vi "总VI.vi"() -> ()   [LabVIEW 2020]
panel:
  out "当前输入/结果":string="0"
  out "历史记录":string
  in  "=":bool
  in  ".":bool
  in  "0":bool
  in  "+/-":bool
  in  "+":bool
  in  "3":bool
  in  "2":bool
  in  "1":bool
  in  "-":bool
  in  "6":bool
  in  "5":bool
  in  "4":bool
  in  "*":bool
  in  "9":bool
  in  "8":bool
  in  "7":bool
  in  "/":bool
  in  "平方根":bool
  in  "x^2":bool
  in  "1/x":bool
  in  "回删":bool
  in  "清空全部":bool
  in  "清除输入":bool
  in  "%":bool
  # "标准"
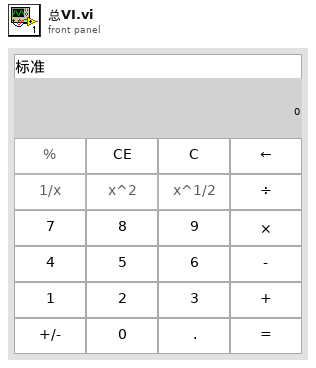
[diagram p1: front panel]
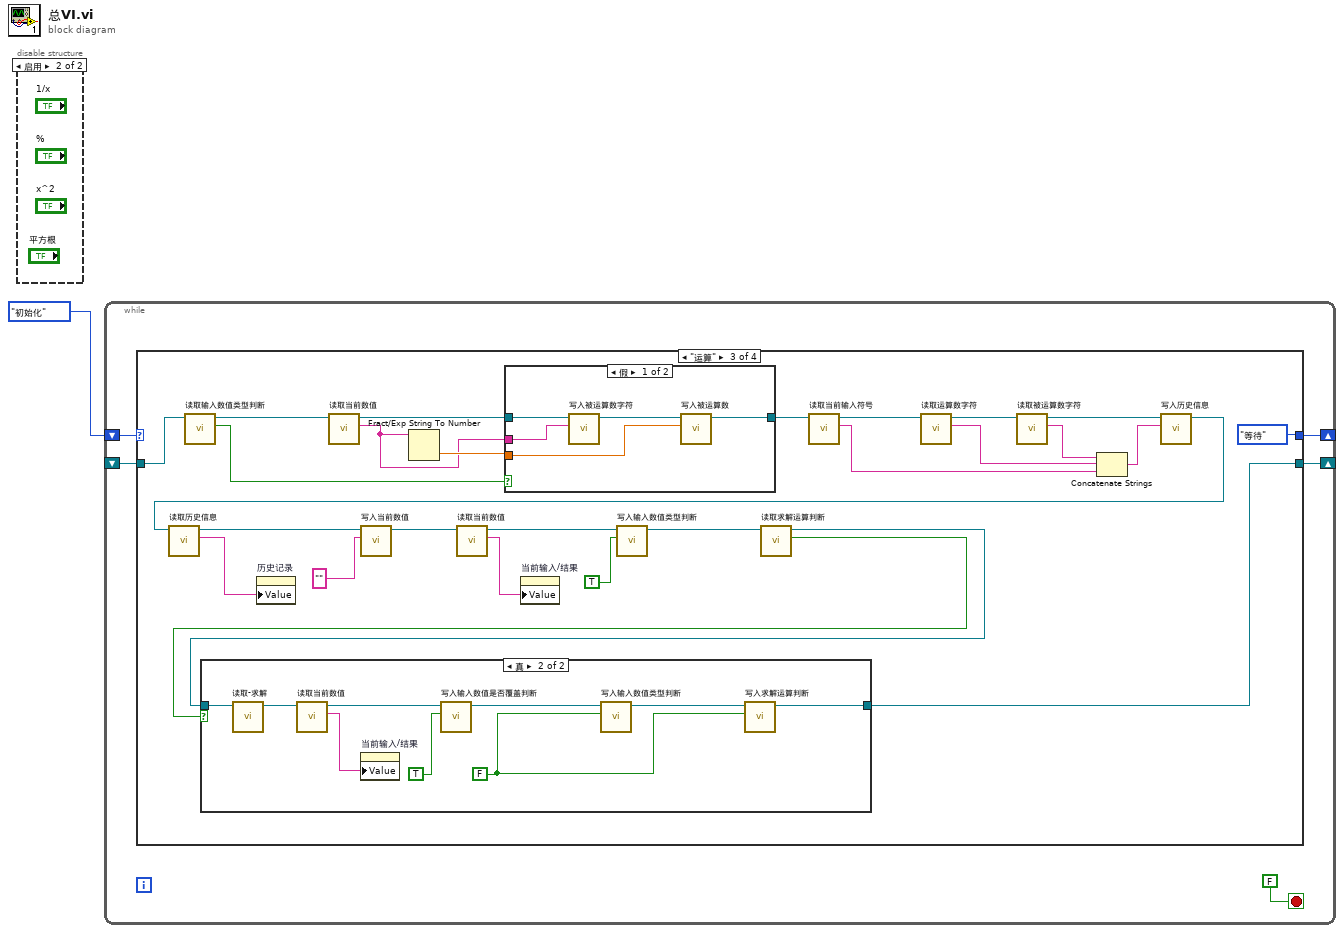
[diagram p0: block diagram]
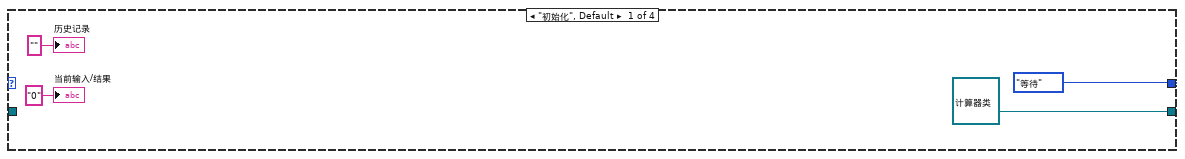
[diagram p2: hidden frame]
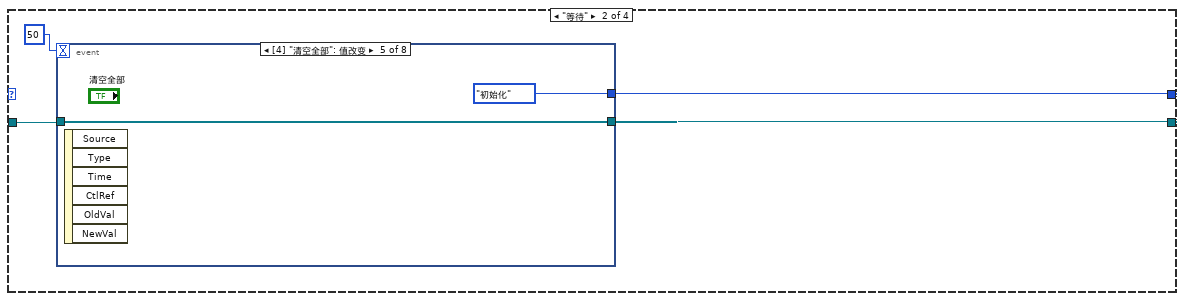
[diagram p3: hidden frame]
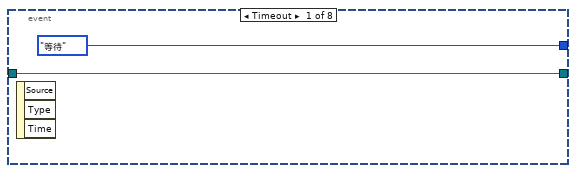
[diagram p4: hidden frame]
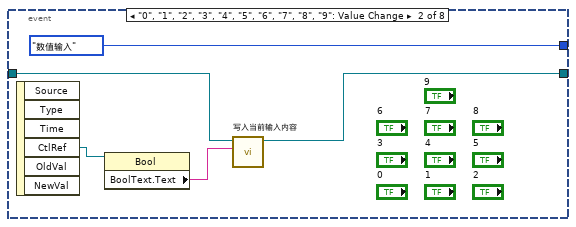
[diagram p5: hidden frame]
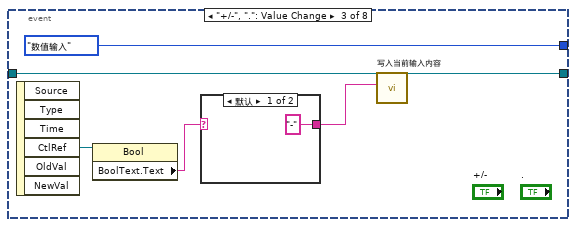
[diagram p6: hidden frame]
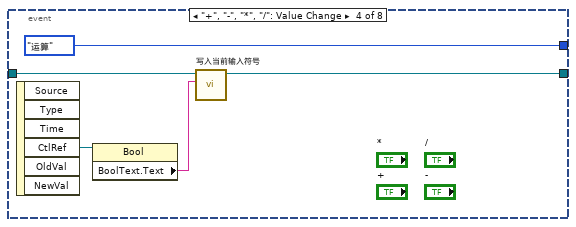
[diagram p8: hidden frame]
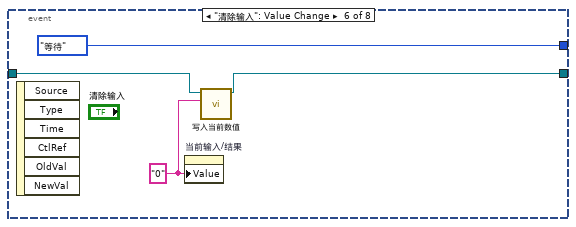
[diagram p9: hidden frame]
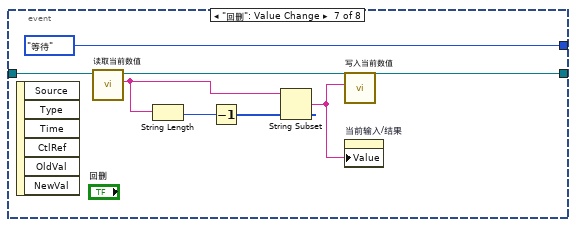
[diagram p10: hidden frame]
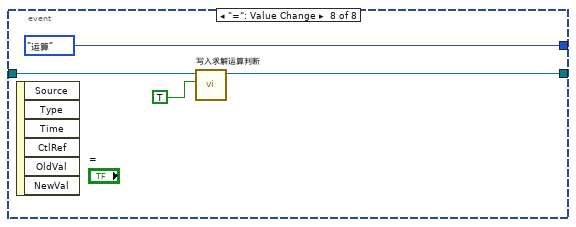
[diagram p11: hidden frame]
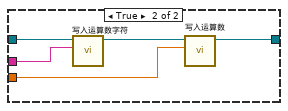
[diagram p13: hidden frame]
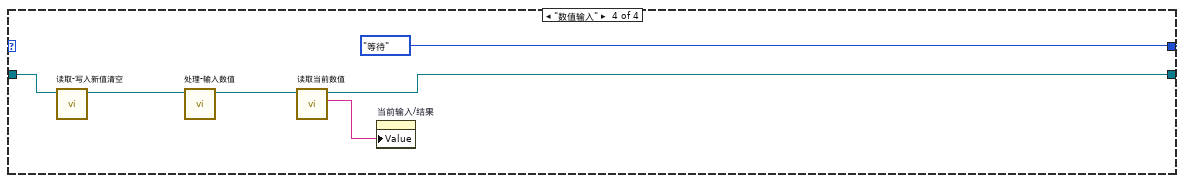
[diagram p14: hidden frame]
diagram:
  n1 = disable-structure shown="启用" {
    frame Disabled {
    }
    frame Enabled {
    }
  }
  n2 = while {
    shift-right: [w4] -> _
    shift-left: enum16{"初始化", "等待", "运算", "数值输入"}."初始化" -> [w5]
    shift-right: [w3] -> _
    shift-left: _ -> [w2]
    stop <- FALSE stop-if-true
    n3 = case shown="\"运算\"" w5 {
      tunnel: [enum16{"初始化", "等待", "运算", "数值输入"}."等待" w14 enum16{"初始化", "等待", "运算", "数值输入"}."等待" enum16{"初始化", "等待", "运算", "数值输入"}."等待"] -> w4
      tunnel: [refnum<class "计算器类.lvclass"> refnum ("计算器类.lvclass") w11 w76 w102] -> w3
      tunnel: w2 -> [_ w12 w77 w104]
      frame "初始化", Default {
        "历史记录" <- "" ("历史记录")
        "当前输入/结果" <- "0" ("当前输入/结果")
      }
      frame "等待" {
        n4 = event shown="[4] \"清空全部\": 值改变" {
          selector: _ -> [_ _ _ _ _ _ _ _]
          dyn-events: _ -> [_ _ _ _ _ _ _ _]
          timeout: 50 -> [_ _ _ _ _ _ _ _]
          tunnel: [enum16{"初始化", "等待", "运算", "数值输入"}."等待" enum16{"初始化", "等待", "运算", "数值输入"}."数值输入" enum16{"初始化", "等待", "运算", "数值输入"}."数值输入" enum16{"初始化", "等待", "运算", "数值输入"}."运算" enum16{"初始化", "等待", "运算", "数值输入"}."初始化" enum16{"初始化", "等待", "运算", "数值输入"}."等待" enum16{"初始化", "等待", "运算", "数值输入"}."等待" enum16{"初始化", "等待", "运算", "数值输入"}."运算"] -> w14
          tunnel: w12 -> [w16 w19 w24 w32 w35 w40 w42 w52]
          tunnel: [w16 w18 w23 w31 w35 w38 w45 w50] -> w11
          event Timeout {
            n5 = event-data() -> ()  [unwired: 1 in, 3 out]
          }
          event "0", "1", "2", "3", "4", "5", "6", "7", "8", "9": Value Change {
            n6 = event-data() -> ("CtlRef"=w21:refnum<vi>)  [unwired: 1 in, 5 out]
            n7 = property class="Bool"(reference=w21) -> ("BoolText.Text"=w20:string)  [unwired: 1 in, 2 out]
            n8 = call "写入当前输入内容.vi"("当前输入内容"=w20, "计算器类输入"=w19) -> ("计算器类输出"=w18:refnum<class "计算器类.lvclass">)  [unwired: 8 in, 1 out]
          }
          event "+/-", ".": Value Change {
            n9 = event-data() -> ("CtlRef"=w27:refnum<vi>)  [unwired: 1 in, 5 out]
            n10 = property class="Bool"(reference=w27) -> ("BoolText.Text"=w26:string)  [unwired: 1 in, 2 out]
            n11 = case shown="默认" w26 {
              selector: w26 -> [_ w29]
              tunnel: ["-" w29] -> w25
              frame Default {
              }
              frame "." {
              }
            }
            n12 = call "写入当前输入内容.vi"("当前输入内容"=w25, "计算器类输入"=w24) -> ("计算器类输出"=w23:refnum<class "计算器类.lvclass">)  [unwired: 8 in, 1 out]
          }
          event "+", "-", "*", "/": Value Change {
            n13 = event-data() -> ("CtlRef"=w34:refnum<vi>)  [unwired: 1 in, 5 out]
            n14 = property class="Bool"(reference=w34) -> ("BoolText.Text"=w33:string)  [unwired: 1 in, 2 out]
            n15 = call "写入当前输入符号.vi"("当前输入符号"=w33, "计算器类输入"=w32) -> ("计算器类输出"=w31:refnum<class "计算器类.lvclass">)  [unwired: 8 in, 1 out]
          }
          event "清空全部": Value Change {
            n16 = event-data() -> ()  [unwired: 1 in, 6 out]
          }
          event "清除输入": Value Change {
            w39 = "0" ("当前输入/结果")
            n17 = event-data() -> ()  [unwired: 1 in, 6 out]
            n18 = property on="当前输入/结果" class="Str"("Value"=w39) -> ()  [unwired: 2 in, 2 out]
            n19 = call "写入当前数值.vi"("当前数值"=w39, "计算器类输入"=w40) -> ("计算器类输出"=w38:refnum<class "计算器类.lvclass">)  [unwired: 8 in, 1 out]
          }
          event "回删": Value Change {
            n20 = event-data() -> ()  [unwired: 1 in, 6 out]
            n21 = call "读取当前数值.vi"("计算器类输入"=w42) -> ("当前数值"=w44:string, "计算器类输出"=w43:refnum<class "计算器类.lvclass">)  [unwired: 8 in, 1 out]
            n22 = String Length(string=w44) -> (length=w48:i32)
            n23 = Decrement(x=w48) -> (x-1=w47:i32)
            n24 = String Subset(string=w44, length (rest)=w47) -> (substring=w46:string)  [unwired: 1 in]
            n25 = call "写入当前数值.vi"("当前数值"=w46, "计算器类输入"=w43) -> ("计算器类输出"=w45:refnum<class "计算器类.lvclass">)  [unwired: 8 in, 1 out]
            n26 = property on="当前输入/结果" class="Str"("Value"=w46) -> ()  [unwired: 2 in, 2 out]
          }
          event "=": Value Change {
            n27 = event-data() -> ()  [unwired: 1 in, 6 out]
            n28 = call "写入求解运算判断.vi"("求解运算判断"=TRUE ("求解判断"), "计算器类输入"=w52) -> ("计算器类输出"=w50:refnum<class "计算器类.lvclass">)  [unwired: 8 in, 1 out]
          }
        }
      }
      frame "运算" {
        n29 = call "读取输入数值类型判断.vi"("计算器类输入"=w77) -> ("输入数值类型判断"=w71:bool, "计算器类输出"=w70:refnum<class "计算器类.lvclass">)  [unwired: 8 in, 1 out]
        n30 = call "读取当前数值.vi"("计算器类输入"=w70) -> ("当前数值"=w73:string, "计算器类输出"=w72:refnum<class "计算器类.lvclass">)  [unwired: 8 in, 1 out]
        n31 = Fract/Exp String To Number(string=w73) -> (number=w74:dbl)  [unwired: 3 in, 1 out]
        n32 = case shown="假" w71 {
          tunnel: w74 -> [w91 w97]
          tunnel: w73 -> [w93 w99]
          tunnel: w72 -> [w94 w98]
          tunnel: [w90 w95] -> w79
          frame False {
            n33 = call "写入被运算数字符.vi"("被运算数字符"=w93, "计算器类输入"=w94) -> ("计算器类输出"=w92:refnum<class "计算器类.lvclass">)  [unwired: 8 in, 1 out]
            n34 = call "写入被运算数.vi"("被运算数"=w91, "计算器类输入"=w92) -> ("计算器类输出"=w90:refnum<class "计算器类.lvclass">)  [unwired: 8 in, 1 out]
          }
          frame True {
            n35 = call "写入运算数字符.vi"("运算数字符"=w99, "计算器类输入"=w98) -> ("计算器类输出"=w96:refnum<class "计算器类.lvclass">)  [unwired: 8 in, 1 out]
            n36 = call "写入运算数.vi"("运算数"=w97, "计算器类输入"=w96) -> ("计算器类输出"=w95:refnum<class "计算器类.lvclass">)  [unwired: 8 in, 1 out]
          }
        }
        n37 = call "读取当前输入符号.vi"("计算器类输入"=w79) -> ("当前输入符号"=w69:string, "计算器类输出"=w55:refnum<class "计算器类.lvclass">)  [unwired: 8 in, 1 out]
        n38 = call "读取运算数字符.vi"("计算器类输入"=w55) -> ("运算数字符"=w68:string, "计算器类输出"=w54:refnum<class "计算器类.lvclass">)  [unwired: 8 in, 1 out]
        n39 = call "读取被运算数字符.vi"("计算器类输入"=w54) -> ("被运算数字符"=w58:string, "计算器类输出"=w53:refnum<class "计算器类.lvclass">)  [unwired: 8 in, 1 out]
        n40 = Concatenate Strings(w58, w69, w68) -> (w67:string)
        n41 = call "写入历史信息.vi"("历史信息"=w67, "计算器类输入"=w53) -> ("计算器类输出"=w66:refnum<class "计算器类.lvclass">)  [unwired: 8 in, 1 out]
        n42 = call "读取历史信息.vi"("计算器类输入"=w66) -> ("历史信息"=w65:string, "计算器类输出"=w64:refnum<class "计算器类.lvclass">)  [unwired: 8 in, 1 out]
        n43 = property on="历史记录" class="Str"("Value"=w65) -> ()  [unwired: 2 in, 2 out]
        n44 = call "写入当前数值.vi"("当前数值"="" ("当前输入/结果"), "计算器类输入"=w64) -> ("计算器类输出"=w62:refnum<class "计算器类.lvclass">)  [unwired: 8 in, 1 out]
        n45 = call "读取当前数值.vi"("计算器类输入"=w62) -> ("当前数值"=w61:string, "计算器类输出"=w59:refnum<class "计算器类.lvclass">)  [unwired: 8 in, 1 out]
        n46 = property on="当前输入/结果" class="Str"("Value"=w61) -> ()  [unwired: 2 in, 2 out]
        n47 = call "写入输入数值类型判断.vi"("输入数值类型判断"=TRUE ("运算符判断"), "计算器类输入"=w59) -> ("计算器类输出"=w78:refnum<class "计算器类.lvclass">)  [unwired: 8 in, 1 out]
        n48 = call "读取求解运算判断.vi"("计算器类输入"=w78) -> ("求解运算判断"=w57:bool, "计算器类输出"=w56:refnum<class "计算器类.lvclass">)  [unwired: 8 in, 1 out]
        n49 = case shown="真" w57 {
          tunnel: w56 -> [w80 w87]
          tunnel: [w80 w81] -> w76
          frame False {
          }
          frame True {
            w82 = FALSE ("运算符判断")
            n50 = call "读取-求解.vi"("计算器类 输入"=w87) -> ("计算器类 输出"=w89:refnum<class "计算器类.lvclass">)  [unwired: 9 in, 1 out]
            n51 = call "读取当前数值.vi"("计算器类输入"=w89) -> ("当前数值"=w88:string, "计算器类输出"=w85:refnum<class "计算器类.lvclass">)  [unwired: 8 in, 1 out]
            n52 = property on="当前输入/结果" class="Str"("Value"=w88) -> ()  [unwired: 2 in, 2 out]
            n53 = call "写入输入数值是否覆盖判断.vi"("输入数值是否覆盖判断"=TRUE ("输入值操作判断"), "计算器类输入"=w85) -> ("计算器类输出"=w84:refnum<class "计算器类.lvclass">)  [unwired: 8 in, 1 out]
            n54 = call "写入输入数值类型判断.vi"("输入数值类型判断"=w82, "计算器类输入"=w84) -> ("计算器类输出"=w83:refnum<class "计算器类.lvclass">)  [unwired: 8 in, 1 out]
            n55 = call "写入求解运算判断.vi"("求解运算判断"=w82, "计算器类输入"=w83) -> ("计算器类输出"=w81:refnum<class "计算器类.lvclass">)  [unwired: 8 in, 1 out]
          }
        }
      }
      frame "数值输入" {
        n56 = call "读取-写入新值清空.vi"("计算器类 输入"=w104) -> ("计算器类 输出"=w103:refnum<class "计算器类.lvclass">)  [unwired: 9 in, 1 out]
        n57 = call "处理-输入数值.vi"("计算器类 输入"=w103) -> ("计算器类 输出"=w101:refnum<class "计算器类.lvclass">)  [unwired: 9 in, 1 out]
        n58 = call "读取当前数值.vi"("计算器类输入"=w101) -> ("当前数值"=w100:string, "计算器类输出"=w102:refnum<class "计算器类.lvclass">)  [unwired: 8 in, 1 out]
        n59 = property on="当前输入/结果" class="Str"("Value"=w100) -> ()  [unwired: 2 in, 2 out]
      }
    }
  }
